vi "Player Info.vi"(11 "Formation in":refnum<class "Formation.lvclass">) -> (1 "Victory Speech":string, 2 "Name":string, 3 "Formation out":refnum<class "Formation.lvclass">)   [LabVIEW 2015, in "Formation.lvclass"]
uses:
  Formation.lvclass
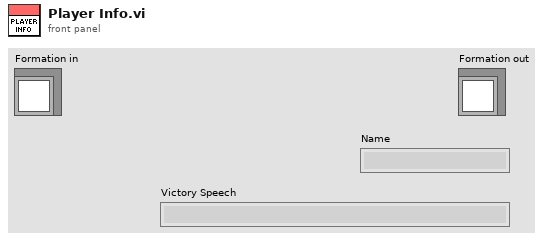
[diagram p1: front panel]
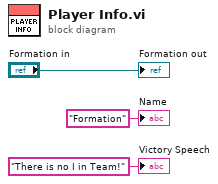
[diagram p0: block diagram]
diagram:
  "Formation out" <- "Formation in"
  "Name" <- "Formation" ("Name")
  "Victory Speech" <- "There is no I in Team!" ("Victory Speech")
